vi "SV Histogram from Buffered Data (1 Ch) (DBL).vi"(0 "new data":dbl[](array[numeric]), 1 "reset (F)":bool, 5 "range":cluster{"minimum":dbl, "maximum":dbl}={"minimum"=-10.0, "maximum"=10.0}, 7 "number of bins (20)":i32=20) -> (4 "histogram":cluster{"bin centers":dbl[], "counts":u64[]}(graph), 6 "actual range":cluster{"minimum":dbl, "maximum":dbl}={"minimum"=-10.0, "maximum"=10.0}, 8 "counts":T1)   [LabVIEW 2017]
doc: "Use this VI to create a histogram of the input data. Set <B>range</B> and <B>number of bins</B> to specify the bins to include. Choose the appropriate instance based on the input data."
uses:
  <vilib>/addons/_NISVFA/_Shared subVIs/Controls/svc_Histogram Counts.ctl
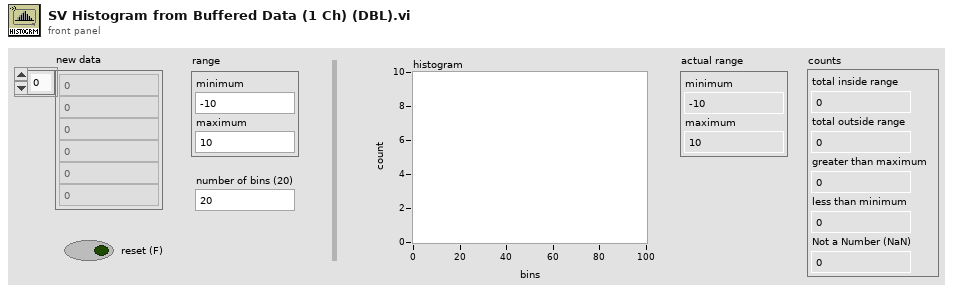
[diagram p1: front panel]
types:
  T1 = typedef "svc_Histogram Counts.ctl" = cluster{"total inside range":u64, "total outside range":u64, "greater than maximum":u64, "less than minimum":u64, "Not a Number (NaN)":u64}
  T2 = typedef "svc_Bin Specification.ctl" = cluster{"lower":dbl, "upper":dbl, "inclusion":u32}
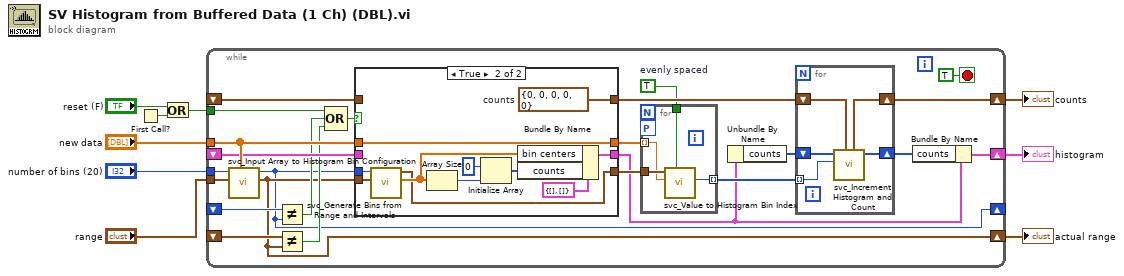
[diagram p0: block diagram]
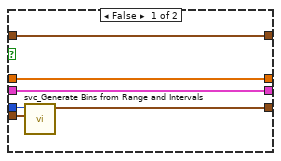
[diagram p2: hidden frame]
diagram:
  n1 = First Call?() -> (First Call?: T/F=w5:bool)
  n2 = Or(x="reset (F)", y=w5) -> (x .or. y?=w4:bool)
  n3 = while {
    tunnel: "new data" -> [w25]
    shift-right: [w30] -> w7
    shift-left: _ -> [w28]
    shift-right: [w33] -> w9
    shift-left: _ -> [w22]
    tunnel: w4 -> [w14]
    tunnel: "number of bins (20)" -> [w26]
    tunnel: "range" -> [w24]
    shift-right: [w11] -> w1
    shift-left: _ -> [w21]
    shift-right: [w10] -> _
    shift-left: _ -> [w23]
    stop <- TRUE stop-if-true
    w20 = TRUE  # evenly spaced
    n4 = call <vilib>:"svc_Input Array to Histogram Bin Configuration.vi"("input data"=w25, "range in"=w24, "number of bins in"=w26) -> ("range out"=w11:cluster{"minimum":dbl, "maximum":dbl}, "number of bins out"=w10:i32)  [unwired: 7 in]
    n5 = Not Equal?(x=w23, y=w10) -> (x != y?=w16:bool)
    n6 = Not Equal?(x=w21, y=w11) -> (x != y?=w15:bool)
    n7 = Compound Arithmetic op=OR(w14, w16, w15) -> (w13:bool)
    n8 = case shown="True" w13 {
      tunnel: [w39 w50] -> w29
      tunnel: w28 -> [w39 _]
      tunnel: w25 -> [w38 w49]
      tunnel: [w38 w49] -> w27
      tunnel: w10 -> [w36 w47]
      tunnel: w11 -> [w37 w46]
      tunnel: w22 -> [w35 _]
      tunnel: [w34 w41] -> w19
      tunnel: [w35 w44] -> w17
      frame False {
        n9 = call <vilib>:"svc_Generate Bins from Range and Intervals.vi"("range"=w37, "number of bins"=w36) -> ("bins"=w34:T2[])  [unwired: 8 in, 1 out]
      }
      frame True {
        w50 = T1 {"total inside range"=0, "total outside range"=0, "greater than maximum"=0, "less than minimum"=0, "Not a Number (NaN)"=0}  # counts
        n10 = call <vilib>:"svc_Generate Bins from Range and Intervals.vi"("range"=w46, "number of bins"=w47) -> ("nominal centers"=w43:dbl[], "bins"=w41:T2[])  [unwired: 8 in]
        n11 = Array Size(array=w43) -> (size(s)=w42:i32)
        n12 = Initialize Array(u64 0 ("element"), w42) -> (w40:u64[])
        n13 = Bundle By Name(cluster=cluster{"bin centers":dbl[], "counts":u64[]} {"bin centers"=[], "counts"=[]}, "bin centers"=w43, "counts"=w40) -> (w44:cluster{"bin centers":dbl[], "counts":u64[]})
      }
    }
    n14 = for {
      tunnel: w27 -> [w53] mode=indexing
      tunnel: [w52] -> w31 mode=indexing
      workers-P: _ -> [_]
      tunnel: w19 -> [w54]
      tunnel: w20 -> [w51]
      n15 = call <vilib>:"svc_Value to Histogram Bin Index.vi"("evenly spaced (F)"=w51, "value"=w53, "bins in"=w54) -> ("bin index"=w52:i32)  [unwired: 7 in, 1 out]
    }
    n16 = Unbundle By Name(w17) -> ("counts"=w18:u64[])
    n17 = for {
      shift-right: [w56] -> w32
      shift-left: w18 -> [w57]
      shift-right: [w58] -> w30
      shift-left: w29 -> [w59]
      tunnel: w31 -> [w55] mode=indexing
      n18 = call <vilib>:"svc_Increment Histogram and Count.vi"("counts in"=w59, "bin index"=w55, "histogram in"=w57) -> ("histogram out"=w56:u64[], "counts out"=w58:T1)  [unwired: 7 in]
    }
    n19 = Bundle By Name(cluster=w17, "counts"=w32) -> (w33:cluster{"bin centers":dbl[], "counts":u64[]})
  }
  "counts" <- w7
  "histogram" <- w9
  "actual range" <- w1
